vi "16 BIT Register.vi"(1 "Clock":bool, 2 "Data In":bool[](array[boolean])=[FALSE, FALSE, FALSE, FALSE, FALSE, FALSE, FALSE, FALSE, FALSE, FALSE, FALSE, FALSE, FALSE, FALSE, FALSE, FALSE], 3 "Hold":bool) -> (0 "Data Out":bool[](array[boolean]))   [LabVIEW 2012]
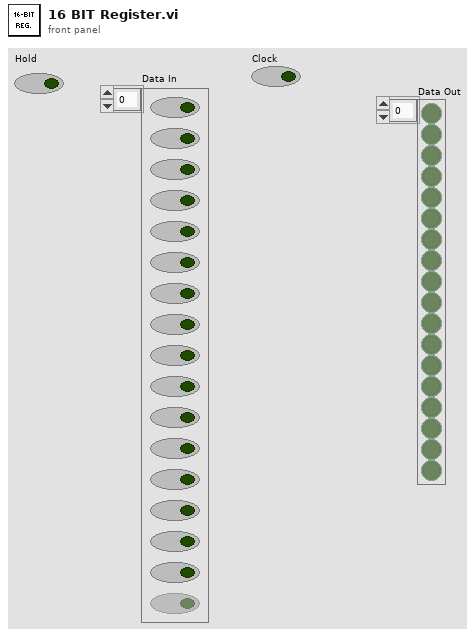
[diagram p1: front panel]
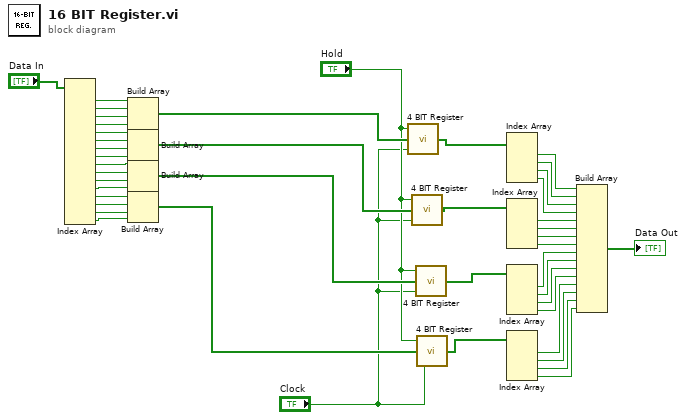
[diagram p0: block diagram]
diagram:
  n1 = Index Array(array="Data In") -> (element #1=w44:bool, element #2=w43:bool, element #3=w42:bool, element #4=w41:bool, element #5=w40:bool, element #6=w39:bool, element #7=w38:bool, element #8=w37:bool, element #9=w36:bool, element #10=w35:bool, element #11=w34:bool, element #12=w33:bool, element #13=w32:bool, element #14=w31:bool, element #15=w30:bool, element #16=w29:bool)  [unwired: 16 in]
  n2 = Build Array(w44, w43, w42, w41) -> (w4:bool[])
  n3 = Build Array(w40, w39, w38, w37) -> (w5:bool[])
  n4 = Build Array(w36, w35, w34, w33) -> (w6:bool[])
  n5 = Build Array(w32, w31, w30, w29) -> (w7:bool[])
  n6 = call "4 BIT Register.vi"("Clock"="Clock", "Data In"=w4, "Hold"="Hold") -> ("Data Out"=w11:bool[])
  n7 = call "4 BIT Register.vi"("Clock"="Clock", "Data In"=w5, "Hold"="Hold") -> ("Data Out"=w10:bool[])
  n8 = call "4 BIT Register.vi"("Clock"="Clock", "Data In"=w6, "Hold"="Hold") -> ("Data Out"=w9:bool[])
  n9 = call "4 BIT Register.vi"("Clock"="Clock", "Data In"=w7, "Hold"="Hold") -> ("Data Out"=w8:bool[])
  n10 = Index Array(array=w11) -> (element #1=w28:bool, element #2=w27:bool, element #3=w26:bool, element #4=w25:bool)  [unwired: 4 in]
  n11 = Index Array(array=w10) -> (element #1=w24:bool, element #2=w23:bool, element #3=w22:bool, element #4=w21:bool)  [unwired: 4 in]
  n12 = Index Array(array=w9) -> (element #1=w20:bool, element #2=w19:bool, element #3=w18:bool, element #4=w17:bool)  [unwired: 4 in]
  n13 = Index Array(array=w8) -> (element #1=w16:bool, element #2=w15:bool, element #3=w14:bool, element #4=w13:bool)  [unwired: 4 in]
  n14 = Build Array(w28, w27, w26, w25, w24, w23, w22, w21, w20, w19, w18, w17, w16, w15, w14, w13) -> (→"Data Out":bool[])
